vi "Configure Trigger Event Blender.vi"(0 "VISA resource name":refnum<visa-resource-name>, 1 "Event ID 3":string, 2 "Event ID 4":string, 5 "Trigger Number (1)":i32=1, 7 "Blender Type (0: And)":i32(ring) items=["And", "Or"], 9 "Event ID 1":string, 11 "error in (no error)":errorcluster, 12 "Event ID 2":string) -> (4 "VISA resource name out":refnum<visa-resource-name>, 15 "error out":errorcluster)   [LabVIEW 2020, in "Keithley 2600 Series.lvlib"]
doc: "Configures the events that trigger the blender.\n\n<b>Note:</b>\nIn order to allow for the configuration to achieve a known default state, it's required to call <b>Reset Trigger Event</b> VI before you call this VI."
uses:
  <instrlib>/Keithley 2600 Series/Keithley 2600 Series.lvlib
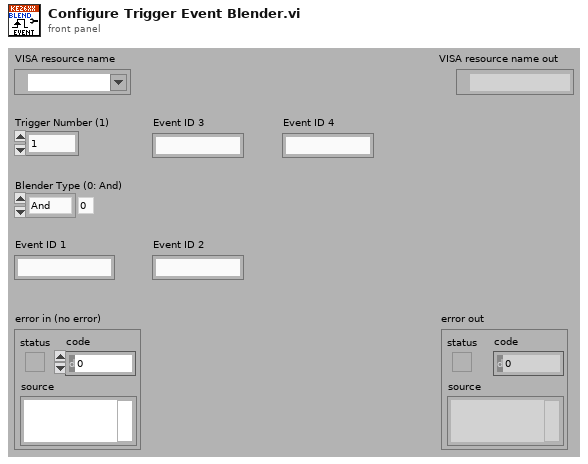
[diagram p1: front panel]
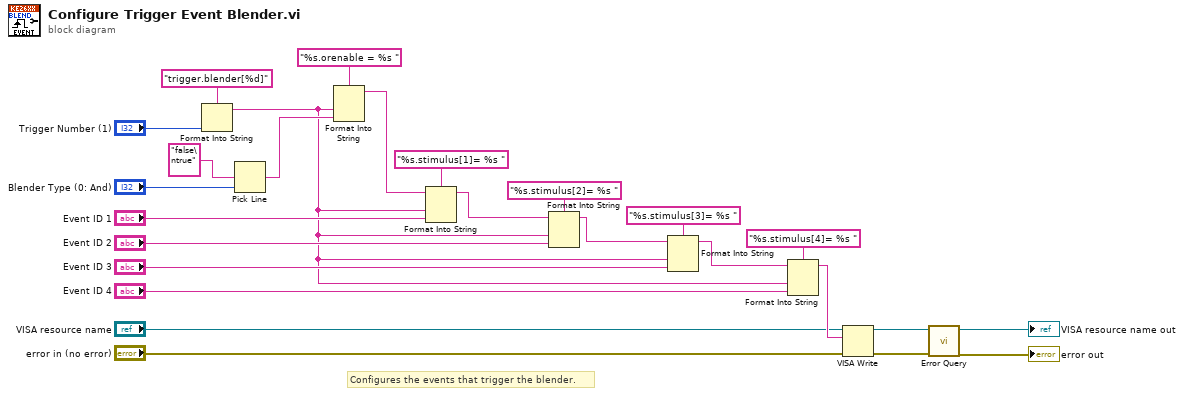
[diagram p0: block diagram]
diagram:
  # "Configures the events that trigger the blender."
  n1 = Format Into String(format string="trigger.blender[%d]", "Trigger Number (1)") -> (resulting string=w5:string)  [unwired: 2 in, 1 out]
  n2 = Pick Line(multi-line string="false\ntrue", line index="Blender Type (0: And)") -> (output string=w20:string)  [unwired: 1 in]
  n3 = Format Into String(format string="%s.orenable = %s ", w5, w20) -> (resulting string=w19:string)  [unwired: 2 in, 1 out]
  n4 = Format Into String(format string="%s.stimulus[1]= %s ", initial string=w19, w5, "Event ID 1") -> (resulting string=w13:string)  [unwired: 1 in, 1 out]
  n5 = Format Into String(format string="%s.stimulus[2]= %s ", initial string=w13, w5, "Event ID 2") -> (resulting string=w12:string)  [unwired: 1 in, 1 out]
  n6 = Format Into String(format string="%s.stimulus[3]= %s ", initial string=w12, w5, "Event ID 3") -> (resulting string=w11:string)  [unwired: 1 in, 1 out]
  n7 = Format Into String(format string="%s.stimulus[4]= %s ", initial string=w11, w5, "Event ID 4") -> (resulting string=w6:string)  [unwired: 1 in, 1 out]
  n8 = VISA Write(VISA resource name="VISA resource name", write buffer=w6, error in (no error)="error in (no error)") -> (VISA resource name out=w2:refnum<visa-resource-name>, error out=w1:errorcluster)  [unwired: 1 out]
  n9 = call <instrlib>:"Error Query.vi"("error in (no error)"=w1, "VISA resource name"=w2) -> ("error out"=→"error out":errorcluster, "VISA resource name out"=→"VISA resource name out":refnum<visa-resource-name>)  [unwired: 6 in, 2 out]
